vi "Cleanup.vi"(8 "error in (no error)":errorcluster, 11 "Start Low Pressure Wax in":refnum<class "Start Low Pressure Wax.lvclass">) -> (0 "error out":errorcluster, 3 "Start Low Pressure Wax out":refnum<class "Start Low Pressure Wax.lvclass">)   [LabVIEW 2019, in "Start Low Pressure Wax.lvclass"]
uses:
  <vilib>/gpm_packages/@cs/Car-wash/Source/Process Steps/Start Low Pressure Wax/Start Low Pressure Wax.lvclass
  <vilib>/gpm_packages/@cs/Car-wash/Source/iProcess Step Model/iProcess Step Model/iProcess Step Model.lvclass
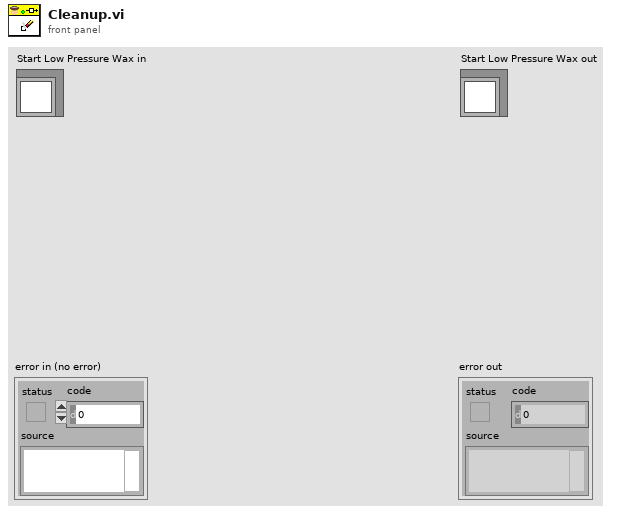
[diagram p1: front panel]
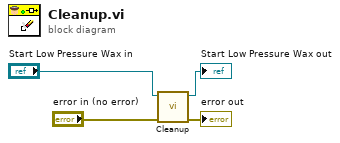
[diagram p0: block diagram]
diagram:
  n1 = call-parent "Cleanup.vi"("error in (no error)"="error in (no error)", "iProcess Step Model in"="Start Low Pressure Wax in") -> ("error out"=→"error out":errorcluster, "iProcess Step Model out"=→"Start Low Pressure Wax out":refnum<class "Start Low Pressure Wax.lvclass">)  [unwired: 8 in]
